vi "GetXml.vi"(8 "error in (no error)":errorcluster, 11 "Project Path":path=path "\\\\vmware-host\\Shared Folders/_Repo/NI-XNET-Monitor-Custom-Device/Source/NI-XNET Monitor Custom Device.lvproj") -> (0 "error out":errorcluster, 2 "XML String":string, 3 "XML Path":path)   [LabVIEW 2020, in "Shared.lvlib"]
uses:
  Shared.lvlib
  <vilib>/xml/Load XML File.vi
  <vilib>/xml/NI_XML.lvlib
  <resource>/objmgr/DOMUserDefRef.rc
  <vilib>/xml/Close Reference(Node).vi
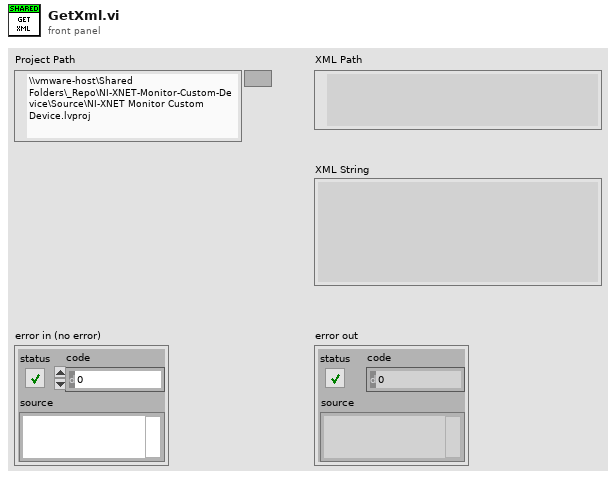
[diagram p1: front panel]
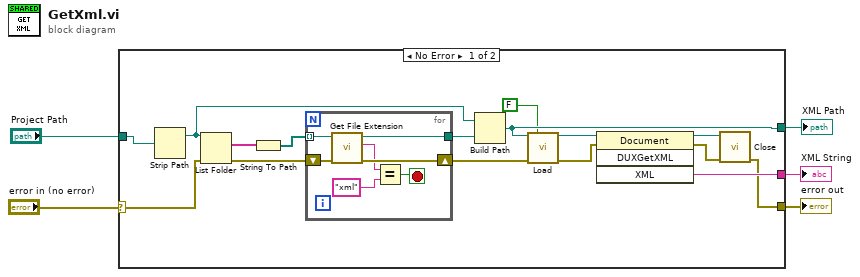
[diagram p0: block diagram]
diagram:
  n1 = case shown="No Error" "error in (no error)" {
    selector: "error in (no error)" -> [w20 w29]
    tunnel: "Project Path" -> [w21 _]
    tunnel: [w6 w29] -> w3
    tunnel: [w12 _] -> w2
    tunnel: [w10 _] -> w1
    frame No Error {
      n2 = Strip Path(path=w21) -> (stripped path=w16:path)  [unwired: 1 out]
      n3 = List Folder(path=w16, error in=w20) -> (filenames=w19:string[], error out=w17:errorcluster)  [unwired: 2 in, 2 out]
      n4 = String To Path(string=w19) -> (path=w18:path[])
      n5 = for {
        tunnel: w18 -> [w28] mode=indexing
        shift-right: [w26] -> w11
        shift-left: w17 -> [w27]
        tunnel: [w22] -> w15
        stop <- w23 stop-if-true
        n6 = call <vilib>:"Get File Extension.vi"("error in (no error)"=w27, "file"=w28) -> ("error out"=w26:errorcluster, "lowercase file extension"=w25:string, "dup file"=w22:path)  [unwired: 5 in, 2 out]
        n7 = Equal?(x=w25, y="xml") -> (x = y?=w23:bool)
      }
      n8 = Build Path(base path=w16, name or relative path=w15) -> (appended path=w10:path)
      n9 = call-poly <vilib>:"Load.vi"("path to XML document"=w10, "preserve whitespace (True)"=FALSE, "error in (no error)"=w11) -> ("DOM document out"=w14:refnum<k20>, "error out"=w13:errorcluster)  [unwired: 10 in, 1 out]
      n10 = invoke class="Document" method="DUXGetXML"(reference=w14, error in=w13) -> (reference out=w8:refnum<k20>, error out=w7:errorcluster, "XML"=w12:string)  [unwired: 2 in, 1 out]
      n11 = call-poly <vilib>:"Close.vi"("error in (no error)"=w7, "node"=w8) -> ("error out"=w6:errorcluster)  [unwired: 7 in]
    }
    frame Error {
    }
  }
  "error out" <- w3
  "XML String" <- w2
  "XML Path" <- w1
